vi "Get Pyramid Vertices.vi"(9 "Type":u16(ring) items=["Triangular", "Square"], 10 "Base":dbl, 11 "Height":dbl) -> (3 "Vertex Array":cluster{"X":dbl, "Y":dbl, "Z":dbl}[](array[cluster]))   [LabVIEW 2023]
doc: "This VI calculates the vertices of a pyramid."
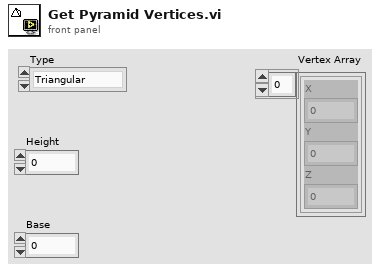
[diagram p1: front panel]
types:
  T1 = cluster{"Height":dbl, "Height":dbl, "Height":dbl}
  T2 = cluster{"Base":dbl, "Height":dbl, "Height":dbl}[]
  T3 = cluster{"Height":dbl, "Height":dbl, "Height":dbl}[]
  T4 = cluster{"Height":dbl, "Base":dbl, "Height":dbl}[]
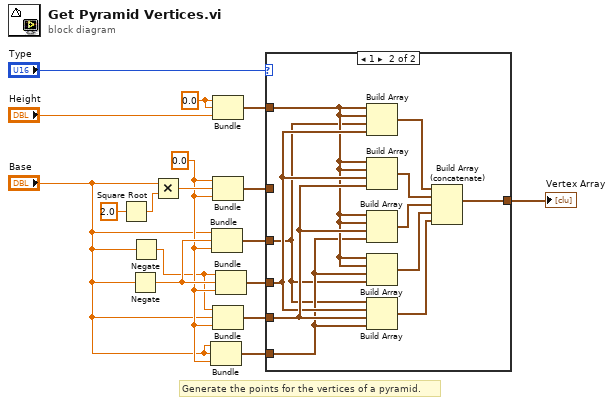
[diagram p0: block diagram]
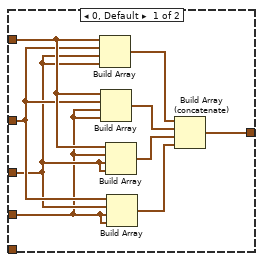
[diagram p2: hidden frame]
diagram:
  w4 = 0.0 ("Height")
  w16 = 0.0 ("Height")
  # "Generate the points for the vertices of a pyramid."
  n1 = Square Root(x=2.0) -> (sqrt(x)=w8:dbl)
  n2 = Negate(x="Base") -> (-x=w6:dbl)
  n3 = Negate(x="Base") -> (-x=w2:dbl)
  n4 = Multiply(x="Base", y=w8) -> (x*y=w10:dbl)
  n5 = Bundle("Base"="Base", "Base"="Base", "Height"=w4) -> (w3:cluster{"Base":dbl, "Base":dbl, "Height":dbl})  [unwired: 1 in]
  n6 = Bundle("Base"="Base", w6, "Height"=w4) -> (w11:cluster{"Base":dbl, dbl, "Height":dbl})  [unwired: 1 in]
  n7 = Bundle("Height"=w16, "Height"=w16, "Height"="Height") -> (w13:T1)  [unwired: 1 in]
  n8 = Bundle("Height"=w4, w10, "Height"=w4) -> (w12:cluster{"Height":dbl, dbl, "Height":dbl})  [unwired: 1 in]
  n9 = Bundle(w2, "Base"="Base", "Height"=w4) -> (w5:cluster{dbl, "Base":dbl, "Height":dbl})  [unwired: 1 in]
  n10 = Bundle(w2, w6, "Height"=w4) -> (w15:cluster{dbl, dbl, "Height":dbl})  [unwired: 1 in]
  n11 = case shown="1" "Type" {
    tunnel: w15 -> [w18 w32]
    tunnel: [w22 w34] -> w14
    tunnel: w13 -> [w21 w29]
    tunnel: w12 -> [w20 _]
    tunnel: w11 -> [w19 w27]
    tunnel: w5 -> [_ w33]
    tunnel: w3 -> [_ w28]
    frame 0, Default {
      n12 = Build Array(w21, w20, w19, w19) -> (w26:T2)
      n13 = Build Array(w21, w20, w18, w18) -> (w25:T3)
      n14 = Build Array(w21, w18, w19, w19) -> (w24:T2)
      n15 = Build Array(w20, w19, w18, w18) -> (w23:cluster{"Base":dbl, dbl, "Height":dbl}[])
      n16 = Build Array (concatenate)(w26, w25, w24, w23) -> (w22:T2)
    }
    frame 1 {
      n17 = Build Array(w29, w29, w27, w32) -> (w37:T2)
      n18 = Build Array(w29, w29, w32, w33) -> (w36:T4)
      n19 = Build Array(w29, w29, w33, w28) -> (w35:cluster{"Base":dbl, "Base":dbl, "Height":dbl}[])
      n20 = Build Array(w29, w29, w28, w27) -> (w31:cluster{"Base":dbl, "Base":dbl, "Height":dbl}[])
      n21 = Build Array(w27, w32, w33, w28) -> (w30:cluster{"Base":dbl, "Base":dbl, "Height":dbl}[])
      n22 = Build Array (concatenate)(w37, w36, w35, w31, w30) -> (w34:cluster{"Base":dbl, "Base":dbl, "Height":dbl}[])
    }
  }
  "Vertex Array" <- w14
